vi "get_number_of_frames.vi"(8 "error in (no error)":errorcluster, 11 "ImagingModeDL100901FlexTrajectory in":refnum<class "ImagingModeDL100901FlexTrajectory.lvclass">) -> (0 "error out":errorcluster, 2 "number of frames":i32, 3 "ImagingModeDL100901FlexTrajectory out":refnum<class "ImagingModeDL100901FlexTrajectory.lvclass">)   [LabVIEW 2010, in "ImagingModeDL100901FlexTrajectory.lvclass"]
uses:
  ImagingModeDL100901FlexTrajectory.lvclass
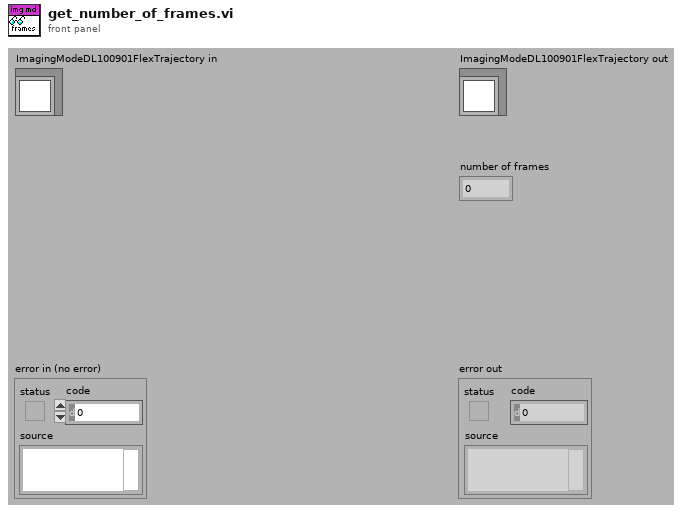
[diagram p1: front panel]
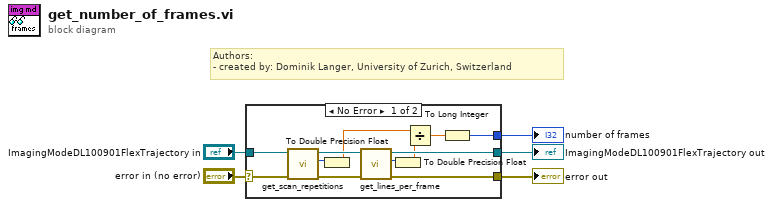
[diagram p0: block diagram]
diagram:
  # "Authors: \n- created by: Dominik Langer, University of Zurich, Switzerland"
  n1 = case shown="No Error" "error in (no error)" {
    selector: "error in (no error)" -> [w15 w19]
    tunnel: [w14 w19] -> w4
    tunnel: [w12 w18] -> w2
    tunnel: "ImagingModeDL100901FlexTrajectory in" -> [w13 w18]
    tunnel: [w6 _] -> w1
    frame No Error {
      n2 = call-dynamic "get_scan_repetitions.vi"("error in (no error)"=w15, "ImagingModeDL100901FlexTrajectory in"=w13) -> ("error out"=w16:errorcluster, "scan repetitions"=w11:i32, "ImagingModeDL100901FlexTrajectory out"=w17:refnum<class "ImagingModeDL100901FlexTrajectory.lvclass">)  [unwired: 7 in]
      n3 = To Double Precision Float(number=w11) -> (double precision float=w10:dbl)
      n4 = call-dynamic "get_lines_per_frame.vi"("error in (no error)"=w16, "ScanModeCN090721ThreeDScan in"=w17) -> ("error out"=w14:errorcluster, "lines per frame"=w9:i32, "ScanModeCN090721ThreeDScan out"=w12:refnum<class "ImagingModeDL100901FlexTrajectory.lvclass">)  [unwired: 7 in]
      n5 = To Double Precision Float(number=w9) -> (double precision float=w8:dbl)
      n6 = Divide(x=w10, y=w8) -> (x/y=w7:dbl)
      n7 = To Long Integer(number=w7) -> (32bit integer=w6:i32)
    }
    frame Error {
    }
  }
  "error out" <- w4
  "ImagingModeDL100901FlexTrajectory out" <- w2
  "number of frames" <- w1
